vi "PointByPointDifference.vi"(7 "reset?":bool=TRUE, 10 "initial condition":dbl, 11 "array":dbl[](array[numeric])) -> (1 "min difference":dbl, 2 "last point":dbl, 3 "max difference":dbl)   [LabVIEW 2017]
panel:
  out "point by point difference":dbl[](array[numeric])
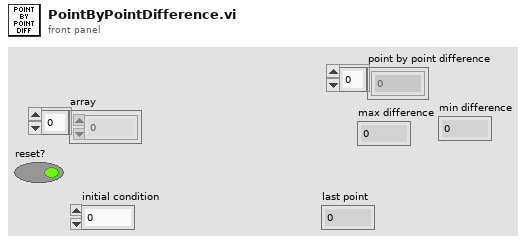
[diagram p1: front panel]
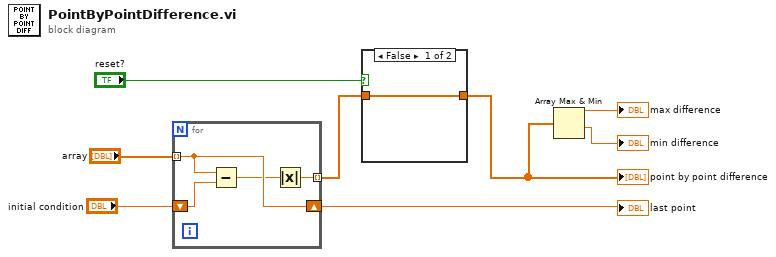
[diagram p0: block diagram]
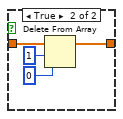
[diagram p2: hidden frame]
diagram:
  n1 = for {
    tunnel: "array" -> [w11] mode=indexing
    shift-right: [w11] -> w6
    shift-left: "initial condition" -> [w12]
    tunnel: [w9] -> w2 mode=indexing
    n2 = Subtract(x=w11, y=w12) -> (x-y=w10:dbl)
    n3 = Absolute Value(x=w10) -> (abs(x)=w9:dbl)
  }
  "last point" <- w6
  n4 = case shown="False" "reset?" {
    tunnel: w2 -> [w13 w17]
    tunnel: [w13 w16] -> w1
    frame False {
    }
    frame True {
      n5 = Delete From Array(array=w17, length=1, index=0) -> (array with subset deleted=w16:dbl[])  [unwired: 1 out]
    }
  }
  "point by point difference" <- w1
  n6 = Array Max & Min(array=w1) -> (max value=→"max difference":dbl, min value=→"min difference":dbl)  [unwired: 2 out]
